vi "Update.vi"(8 "error in (no error)":errorcluster, 10 "Message in":refnum<class "UpdateMessage.lvclass">, 11 "ExampleClassA in":refnum<class "ExampleClassA.lvclass">) -> (0 "error out":errorcluster, 3 "ExampleClassA out":refnum<class "ExampleClassA.lvclass">)   [LabVIEW 2012, in "ExampleClassA.lvclass"]
doc: "Processes the XML settings received via an update message. Upates the settings cluster in the private data accordingly."
uses:
  ExampleClassA.lvclass
  <vilib>/Distrio/Murmex/UpdateMessage/UpdateMessage.lvclass
  ExampleClassA.lvclass/ExampleClassA.ctl
  <vilib>/Distrio/Murmex/Murmex/status_enum.ctl
  <vilib>/Distrio/Murmex/Murmex/Murmex.lvclass
  <vilib>/Distrio/Murmex/Message/Message.lvclass
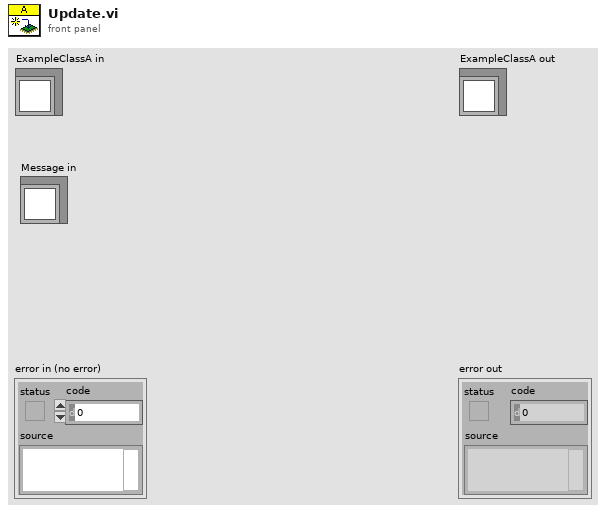
[diagram p1: front panel]
types:
  T1 = typedef "Murmex.lvlib/Murmex.lvclass/status_enum.ctl" = enum16{"ready", "warning", "error", "shutting down", "initialising"}
  T2 = typedef "ExampleClassA.lvclass/Settings cluster.ctl" = cluster{"period?":dbl[unit], "number of blocks":i32, "number of channels":i32}
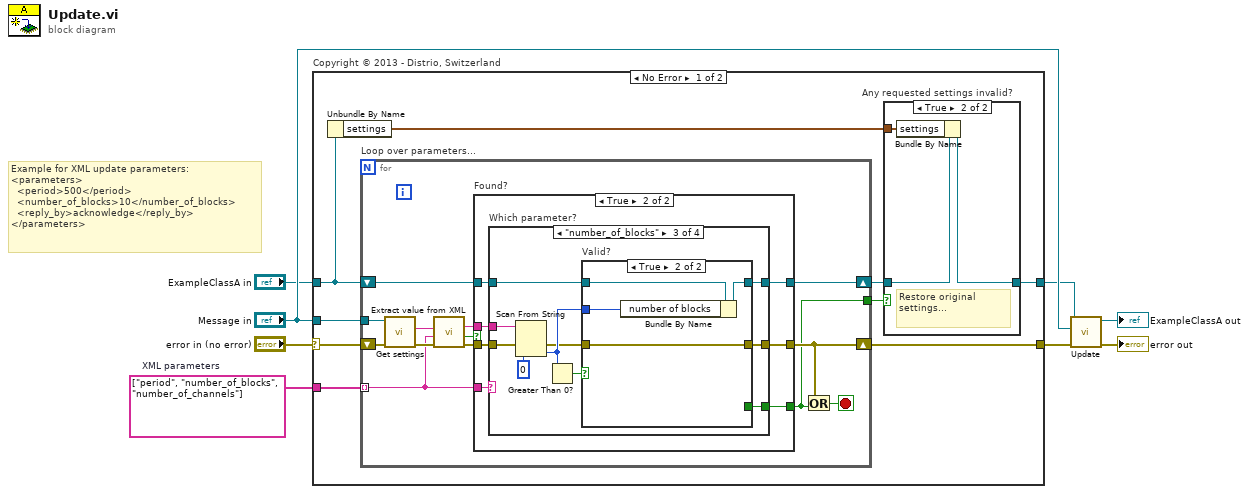
[diagram p0: block diagram]
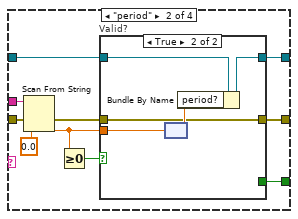
[diagram p5: hidden frame]
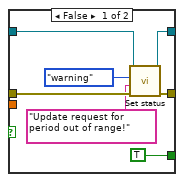
[diagram p6: hidden frame]
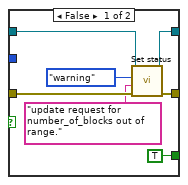
[diagram p7: hidden frame]
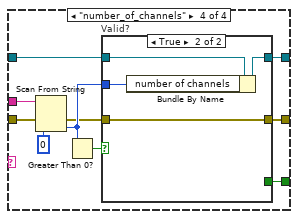
[diagram p8: hidden frame]
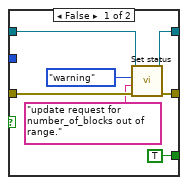
[diagram p9: hidden frame]
diagram:
  w8 = string[] ["period", "number_of_blocks", "number_of_channels"]  # XML parameters
  # "Example for XML update parameters:\n<parameters>\n  <period>500</period>\n  <number_of_blocks>10</number_of_blocks>\n  <reply_by>acknowledge</reply_by>\n</parameters>"
  n1 = case "Copyright © 2013 - Distrio, Switzerland" shown="No Error" "error in (no error)" {
    selector: "error in (no error)" -> [w17 w110]
    tunnel: [w14 w110] -> w7
    tunnel: "ExampleClassA in" -> [w9 w111]
    tunnel: [w10 w111] -> w4
    tunnel: "Message in" -> [w16 _]
    tunnel: w8 -> [w15 _]
    frame No Error {
      n2 = Unbundle By Name(w9) -> ("settings"=w11:T2)
      n3 = for "Loop over parameters..." {
        shift-right: [w32] -> w14
        shift-left: w17 -> [w28]
        tunnel: w15 -> [w25] mode=indexing
        tunnel: w16 -> [w29]
        shift-right: [w33] -> w13
        shift-left: w9 -> [w34]
        tunnel: [w30] -> w12
        stop <- w31 stop-if-true
        n4 = call <vilib>:"Get settings.vi"("error in (no error)"=w28, "UpdateMessage in"=w29) -> ("error out"=w27:errorcluster, "settings"=w26:string)  [unwired: 7 in, 1 out]
        n5 = call <vilib>:"Extract value from XML.vi"("error in (no error)"=w27, "tag name"=w25, "parameters XML"=w26) -> ("error out"=w23:errorcluster, "found?"=w24:bool, "value"=w22:string)  [unwired: 5 in, 1 out]
        n6 = case "Found?" shown="True" w24 {
          tunnel: w23 -> [w36 w40]
          tunnel: [w36 w43] -> w32
          tunnel: w25 -> [_ w42]
          tunnel: w22 -> [_ w41]
          tunnel: w34 -> [w35 w39]
          tunnel: [w35 w38] -> w33
          tunnel: [_ w37] -> w30
          frame False {
          }
          frame True {
            n7 = case "Which parameter?" shown="\"number_of_blocks\"" w42 {
              tunnel: [w45 w47 w70 w91] -> w43
              tunnel: w41 -> [_ w54 w73 w94]
              tunnel: w40 -> [w45 w53 w77 w98]
              tunnel: w39 -> [w44 w52 w75 w96]
              tunnel: [w44 w51 w74 w95] -> w38
              tunnel: [_ w46 w68 w89] -> w37
              frame Default {
              }
              frame "period" {
                n8 = Scan From String(input string=w54, error in=w53, default 1=0.0) -> (error out=w49:errorcluster, output 1=w50:dbl)  [unwired: 2 in, 2 out]
                n9 = Greater Or Equal To 0?(x=w50) -> (x >= 0?=w48:bool)
                n10 = case "Valid?" shown="True" w48 {
                  tunnel: w52 -> [w61 w67]
                  tunnel: [w60 w66] -> w51
                  tunnel: w50 -> [_ w64]
                  tunnel: w49 -> [w62 w63]
                  tunnel: [w59 w63] -> w47
                  tunnel: [TRUE _] -> w46
                  frame False {
                    n11 = call <vilib>:"Set status.vi"("error in (no error)"=w62, "details"="Update request for period out of range!", "status"=status_enum."warning", "Murmex in"=w61) -> ("error out"=w59:errorcluster, "Murmex out"=w60:refnum<class "ExampleClassA.lvclass">)  [unwired: 6 in]
                  }
                  frame True {
                    n12 = node(w64) -> (w65:dbl[unit])
                    n13 = Bundle By Name(cluster=w67, "period?"=w65) -> (w66:refnum<class "ExampleClassA.lvclass">)
                  }
                }
              }
              frame "number_of_blocks" {
                n14 = Scan From String(input string=w73, error in=w77, default 1=0) -> (error out=w71:errorcluster, output 1=w72:i32)  [unwired: 2 in, 2 out]
                n15 = Greater Than 0?(x=w72) -> (x > 0?=w69:bool)
                n16 = case "Valid?" shown="True" w69 {
                  tunnel: w75 -> [w84 w88]
                  tunnel: [w81 w87] -> w74
                  tunnel: w72 -> [_ w86]
                  tunnel: w71 -> [w83 w85]
                  tunnel: [w82 w85] -> w70
                  tunnel: [TRUE _] -> w68
                  frame False {
                    n17 = call <vilib>:"Set status.vi"("error in (no error)"=w83, "details"="update request for number_of_blocks out of range.", "status"=status_enum."warning", "Murmex in"=w84) -> ("error out"=w82:errorcluster, "Murmex out"=w81:refnum<class "ExampleClassA.lvclass">)  [unwired: 6 in]
                  }
                  frame True {
                    n18 = Bundle By Name(cluster=w88, "number of blocks"=w86) -> (w87:refnum<class "ExampleClassA.lvclass">)
                  }
                }
              }
              frame "number_of_channels" {
                n19 = Scan From String(input string=w94, error in=w98, default 1=0) -> (error out=w92:errorcluster, output 1=w93:i32)  [unwired: 2 in, 2 out]
                n20 = Greater Than 0?(x=w93) -> (x > 0?=w90:bool)
                n21 = case "Valid?" shown="True" w90 {
                  tunnel: w96 -> [w105 w109]
                  tunnel: [w102 w108] -> w95
                  tunnel: w93 -> [_ w107]
                  tunnel: w92 -> [w104 w106]
                  tunnel: [w103 w106] -> w91
                  tunnel: [TRUE _] -> w89
                  frame False {
                    n22 = call <vilib>:"Set status.vi"("error in (no error)"=w104, "details"="update request for number_of_blocks out of range.", "status"=status_enum."warning", "Murmex in"=w105) -> ("error out"=w103:errorcluster, "Murmex out"=w102:refnum<class "ExampleClassA.lvclass">)  [unwired: 6 in]
                  }
                  frame True {
                    n23 = Bundle By Name(cluster=w109, "number of channels"=w107) -> (w108:refnum<class "ExampleClassA.lvclass">)
                  }
                }
              }
            }
          }
        }
        n24 = Or(x=w32, y=w30) -> (x .or. y?=w31:bool)
      }
      n25 = case "Any requested settings invalid?" shown="True" w12 {
        tunnel: w13 -> [w18 w21]
        tunnel: w11 -> [_ w20]
        tunnel: [w18 w19] -> w10
        frame False {
        }
        frame True {
          # "Restore original settings..."
          n26 = Bundle By Name(cluster=w21, "settings"=w20) -> (w19:refnum<class "ExampleClassA.lvclass">)
        }
      }
    }
    frame Error {
    }
  }
  n27 = call-parent "Update.vi"("error in (no error)"=w7, "Message in"="Message in", "Murmex in"=w4) -> ("error out"=→"error out":errorcluster, "Murmex out"=→"ExampleClassA out":refnum<class "ExampleClassA.lvclass">)  [unwired: 7 in]
